vi "oa_Compute Cascade Plot Grid Lines.vi"(4 "zoom factor":i32=5, 5 "Y range":cluster{"min":dbl, "max":dbl}={"min"=5.0, "max"=5.0} {"max" format="%.6f"; "min" format="%.6f"}, 6 "plot type":T1(ring), 7 "X scale":cluster{"offset":dbl, "multiplier":dbl} {"multiplier" format="%.2f"; "offset" format="%.2f"}, 8 "Y scale":cluster{"offset":dbl, "multiplier":dbl} {"multiplier" format="%.2f"; "offset" format="%.2f"}, 9 "# of bins":i32, 10 "grid lines to plot [Hz/Order]":dbl[](array[numeric]), 11 "waterfall plot":cluster{"X0":dbl, "dX":dbl, "Y":dbl[]}[](array[cluster]) {"Y" format="%.2f"; "dX" format="%.2f"; "X0" format="%.2f"}) -> (0 "# of axis lines":i32, 1 "# of grid lines":i32, 3 "waterfall plot out":cluster{"X0":dbl, "dX":dbl, "Y":dbl[]}[](array[cluster]) {"Y" format="%.2f"; "dX" format="%.2f"; "X0" format="%.2f"})   [LabVIEW 2017]
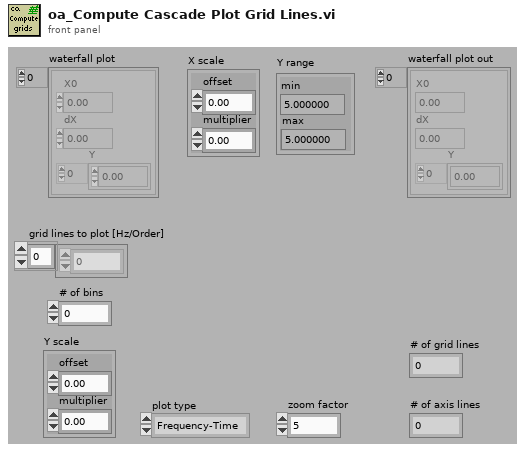
[diagram p1: front panel]
types:
  T1 = enum16{"Frequency-Time", "Time-Frequency", "Order-Time", "Time-Order", "Frequency-RPM", "RPM-Frequency", "Order-RPM", "RPM-Order"}
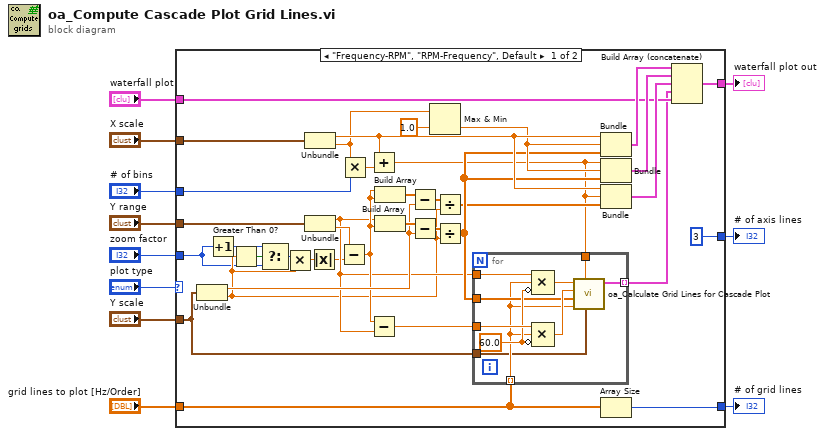
[diagram p0: block diagram]
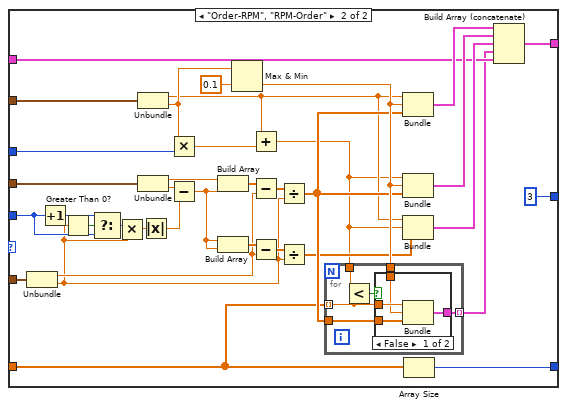
[diagram p2: hidden frame]
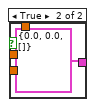
[diagram p3: hidden frame]
diagram:
  n1 = case shown="\"Frequency-RPM\", \"RPM-Frequency\", Default" "plot type" {
    tunnel: "Y range" -> [w43 w94]
    tunnel: "X scale" -> [w44 w93]
    tunnel: "zoom factor" -> [w16 w61]
    tunnel: "waterfall plot" -> [w25 w82]
    tunnel: [w45 w90] -> w7
    tunnel: "# of bins" -> [w40 w88]
    tunnel: "grid lines to plot [Hz/Order]" -> [w37 w67]
    tunnel: [w48 w84] -> w4
    tunnel: "Y scale" -> [w20 w75]
    tunnel: [3 3] -> w1
    frame "Frequency-RPM", "RPM-Frequency", Default {
      n2 = Unbundle(w20) -> ("offset"=w27:dbl, "multiplier"=w18:dbl)
      n3 = Increment(x=w16) -> (x+1=w15:i32)
      n4 = Greater Than 0?(x=w18) -> (x > 0?=w17:bool)
      n5 = Select(t=w15, s=w17, f=w16) -> (s? t:f=w14:i32)
      n6 = Multiply(x=w14, y=w18) -> (x*y=w19:dbl)
      n7 = Unbundle(w44) -> ("offset"=w38:dbl, "multiplier"=w36:dbl)
      n8 = Unbundle(w43) -> ("min"=w22:dbl, "max"=w47:dbl)
      n9 = Absolute Value(x=w19) -> (abs(x)=w13:dbl)
      n10 = Subtract(x=w47, y=w13) -> (x-y=w24:dbl)
      n11 = Multiply(x=w36, y=w40) -> (x*y=w46:dbl)
      n12 = Add(x=w38, y=w46) -> (x+y=w21:dbl)
      n13 = Subtract(x=w24, y=w22) -> (x-y=w23:dbl)
      n14 = Build Array(w24, w24) -> (w28:dbl[])
      n15 = Build Array(w22, w24) -> (w31:dbl[])
      n16 = Subtract(x=w28, y=w27) -> (x-y=w29:dbl[])
      n17 = Subtract(x=w31, y=w27) -> (x-y=w32:dbl[])
      n18 = Max & Min(x=w36, y=1.0) -> (min(x,y)=w34:dbl)  [unwired: 1 out]
      n19 = Divide(x=w29, y=w18) -> (x/y=w26:dbl[])
      n20 = Divide(x=w32, y=w18) -> (x/y=w30:dbl[])
      n21 = for {
        tunnel: w30 -> [w51]
        tunnel: [w55] -> w12 mode=indexing
        tunnel: w37 -> [w50] mode=indexing
        tunnel: w23 -> [w57]
        tunnel: w22 -> [w58]
        tunnel: w21 -> [w54]
        tunnel: w20 -> [w49]
        w56 = 60.0 ("value")
        n22 = Compound Arithmetic op=MULTIPLY(w58, w50, invert w56) -> (w53:dbl)
        n23 = Compound Arithmetic op=MULTIPLY(w57, w50, invert w56) -> (w52:dbl)
        n24 = call <vilib>:"oa_Calculate Grid Lines for Cascade Plot.vi"("Y scale"=w49, "max x axis value"=w54, "order"=w50, "data"=w51, "multiplier"=w52, "start index"=w53) -> ("output grid lines"=w55:cluster{"offset":dbl, dbl, dbl[]})  [unwired: 5 in]
      }
      n25 = Bundle("offset"=w38, w34, w30) -> (w41:cluster{"offset":dbl, dbl, dbl[]})  [unwired: 1 in]
      n26 = Bundle(w21, w34, w30) -> (w42:cluster{dbl, dbl, dbl[]})  [unwired: 1 in]
      n27 = Bundle("offset"=w38, w21, w26) -> (w39:cluster{"offset":dbl, dbl, dbl[]})  [unwired: 1 in]
      n28 = Array Size(array=w37) -> (size(s)=w48:i32)
      n29 = Build Array (concatenate)(w41, w42, w39, w12, w25) -> (w45:cluster{"X0":dbl, "dX":dbl, "Y":dbl[]}[])
    }
    frame "Order-RPM", "RPM-Order" {
      n30 = Unbundle(w75) -> ("offset"=w70:dbl, "multiplier"=w59:dbl)
      n31 = Increment(x=w61) -> (x+1=w63:i32)
      n32 = Greater Than 0?(x=w59) -> (x > 0?=w64:bool)
      n33 = Select(t=w63, s=w64, f=w61) -> (s? t:f=w62:i32)
      n34 = Multiply(x=w62, y=w59) -> (x*y=w65:dbl)
      n35 = Unbundle(w93) -> ("offset"=w68:dbl, "multiplier"=w80:dbl)
      n36 = Unbundle(w94) -> ("min"=w92:dbl, "max"=w89:dbl)
      n37 = Absolute Value(x=w65) -> (abs(x)=w60:dbl)
      n38 = Multiply(x=w80, y=w88) -> (x*y=w87:dbl)
      n39 = Subtract(x=w89, y=w60) -> (x-y=w73:dbl)
      n40 = Build Array(w92, w73) -> (w76:dbl[])
      n41 = Build Array(w73, w73) -> (w71:dbl[])
      n42 = Max & Min(x=w80, y=0.1) -> (min(x,y)=w78:dbl)  [unwired: 1 out]
      n43 = Add(x=w68, y=w87) -> (x+y=w66:dbl)
      n44 = Subtract(x=w76, y=w70) -> (x-y=w77:dbl[])
      n45 = Subtract(x=w71, y=w70) -> (x-y=w72:dbl[])
      n46 = Divide(x=w77, y=w59) -> (x/y=w74:dbl[])
      n47 = Divide(x=w72, y=w59) -> (x/y=w69:dbl[])
      n48 = for {
        tunnel: w67 -> [w96] mode=indexing
        tunnel: w78 -> [w100]
        tunnel: w74 -> [w99]
        tunnel: [w98] -> w81 mode=indexing
        tunnel: w66 -> [w97]
        n49 = Less?(x=w97, y=w96) -> (x < y?=w95:bool)
        n50 = case shown="False" w95 {
          tunnel: w96 -> [w104 _]
          tunnel: w100 -> [w103 _]
          tunnel: w99 -> [w102 _]
          tunnel: [w101 cluster{"Numeric":dbl, dbl, dbl[]} {"Numeric"=0.0, 0.0, []}] -> w98
          frame False {
            n51 = Bundle("Numeric"=w104, w103, w102) -> (w101:cluster{"Numeric":dbl, dbl, dbl[]})  [unwired: 1 in]
          }
          frame True {
          }
        }
      }
      n52 = Bundle("offset"=w68, w78, w74) -> (w91:cluster{"offset":dbl, dbl, dbl[]})  [unwired: 1 in]
      n53 = Bundle(w66, w78, w74) -> (w86:cluster{dbl, dbl, dbl[]})  [unwired: 1 in]
      n54 = Bundle("offset"=w68, w66, w69) -> (w85:cluster{"offset":dbl, dbl, dbl[]})  [unwired: 1 in]
      n55 = Array Size(array=w67) -> (size(s)=w84:i32)
      n56 = Build Array (concatenate)(w91, w86, w85, w81, w82) -> (w90:cluster{"X0":dbl, "dX":dbl, "Y":dbl[]}[])
    }
  }
  "waterfall plot out" <- w7
  "# of grid lines" <- w4
  "# of axis lines" <- w1
